vi "GetSortedPanes.vi"(8 "error in (no error)":errorcluster, 11 "Panes[]":refnum<vi>[](array[refnum])) -> (0 "error out":errorcluster, 3 "Panes":T1)   [LabVIEW 2022 SP3, in "PentaPanesLibrary.lvlib" / "PentaPanes.lvclass"]
uses:
  PentaPanes.lvclass
  PanesCluster.ctl
panel:
  out "Array":string[](array[string])
  out "appended array":refnum<vi>[](array[refnum])
  out "Center Index":i32
  out "Top Index":i32
  out "Bottom Index":i32
  out "Left Index":i32
  out "Right index":i32
  out "Vertical Center of panes":dbl[](array[numeric])
  out "Horizontal Center of pane":dbl[](array[numeric])
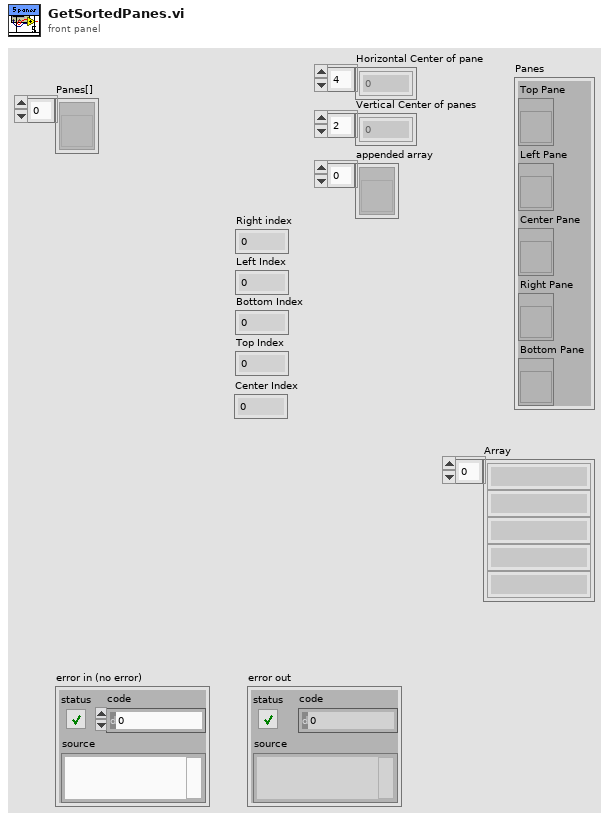
[diagram p1: front panel]
types:
  T1 = typedef "PentaPanesLibrary.lvlib/PentaPanes.lvclass/PanesCluster.ctl" = cluster{"Top Pane":refnum<vi>, "Left Pane":refnum<vi>, "Center Pane":refnum<vi>, "Right Pane":refnum<vi>, "Bottom Pane":refnum<vi>}
  T2 = typedef "LVPointTypeDef.ctl" = cluster{"Horizontal":i16, "Vertical":i16}
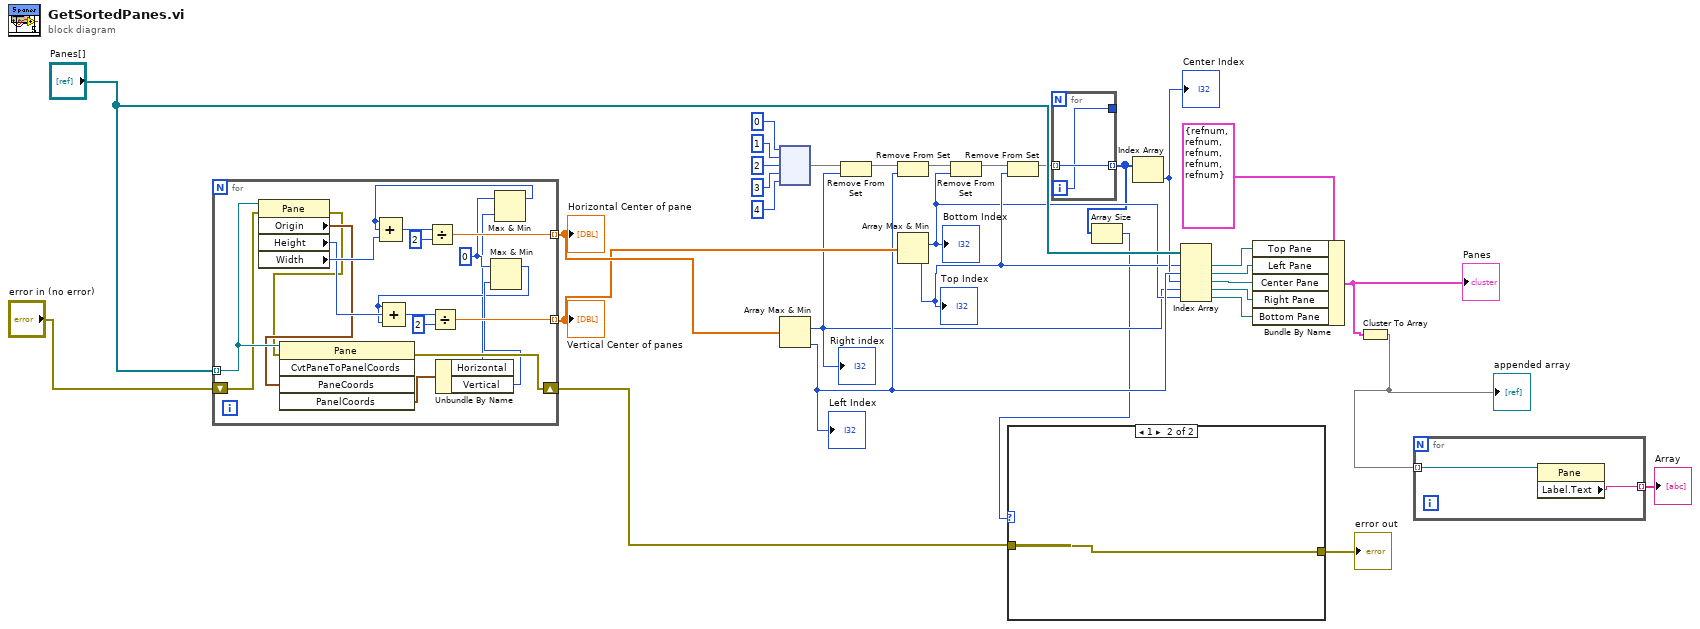
[diagram p0: block diagram]
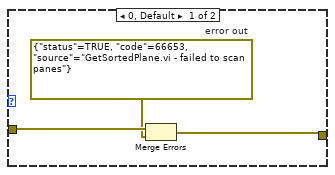
[diagram p2: hidden frame]
diagram:
  n1 = for {
    tunnel: "Panes[]" -> [w43] mode=indexing
    tunnel: [w45] -> w31 mode=indexing
    tunnel: [w44] -> w32 mode=indexing
    shift-right: [w38] -> w3
    shift-left: "error in (no error)" -> [w40]
    w35 = i16 0 ("x")
    n2 = property class="Pane"(reference=w43, error in=w40) -> (error out=w39:errorcluster, "Origin"=w42:T2, "Height"=w46:u32, "Width"=w51:u32)  [unwired: 1 out]
    n3 = invoke class="Pane" method="CvtPaneToPanelCoords"(reference=w43, error in=w39, "PaneCoords"=w42) -> (error out=w38:errorcluster, "PanelCoords"=w41:T2)  [unwired: 2 in, 3 out]
    n4 = Unbundle By Name(w41) -> ("Horizontal"=w34:i16, "Vertical"=w37:i16)
    n5 = Max & Min(x=w35, y=w37) -> (max(x,y)=w36:i16)  [unwired: 1 out]
    n6 = Compound Arithmetic op=ADD(w36, w46, w36) -> (w48:u32)
    n7 = Divide(x=w48, y=u32 2) -> (x/y=w45:dbl)
    n8 = Max & Min(x=w35, y=w34) -> (max(x,y)=w33:i16)  [unwired: 1 out]
    n9 = Compound Arithmetic op=ADD(w33, w33, w51) -> (w50:u32)
    n10 = Divide(x=w50, y=u32 2) -> (x/y=w44:dbl)
  }
  "Horizontal Center of pane" <- w32
  "Vertical Center of panes" <- w31
  n11 = node(0, 1 ("element"), 2 ("element"), 3 ("element"), 4 ("element")) -> (w6:set{i32})
  n12 = Array Max & Min(array=w32) -> (max index (indices)=w7:i32, min index (indices)=w23:i32)  [unwired: 2 out]
  "Right index" <- w7
  "Left Index" <- w23
  n13 = Remove From Set(10:w7, 11:w6) -> (3:w24:set{i32})  [unwired: 1 out]
  n14 = Remove From Set(10:w23, 11:w24) -> (3:w22:set{i32})  [unwired: 1 out]
  n15 = Array Max & Min(array=w31) -> (max index (indices)=w8:i32, min index (indices)=w9:i32)  [unwired: 2 out]
  "Bottom Index" <- w8
  "Top Index" <- w9
  n16 = Remove From Set(10:w8, 11:w22) -> (3:w21:set{i32})  [unwired: 1 out]
  n17 = Remove From Set(10:w9, 11:w21) -> (3:w18:set{i32})  [unwired: 1 out]
  n18 = for {
    tunnel: [w53] -> w5 mode=indexing
    tunnel: w18 -> [w53] mode=indexing
    tunnel: [w52] -> _
    i -> [w52]
  }
  n19 = Array Size(array=w5) -> (size(s)=w4:i32)
  n20 = case shown="1" w4 {
    tunnel: w3 -> [w56 w57]
    tunnel: [w54 w57] -> w2
    frame 0, Default {
      w55 = errorcluster {"status"=TRUE, "code"=66653, "source"="GetSortedPlane.vi - failed to scan panes"}  # error out
      n21 = Merge Errors(w56, w55) -> (w54:errorcluster)
    }
    frame 1 {
    }
  }
  "error out" <- w2
  n22 = Index Array(array=w5) -> (element=w20:i32)  [unwired: 1 in]
  "Center Index" <- w20
  n23 = Index Array(array="Panes[]", index #1=w9, index #2=w23, index #3=w20, index #4=w7, index #5=w8) -> (element #1=w16:refnum<vi>, element #2=w15:refnum<vi>, element #3=w14:refnum<vi>, element #4=w13:refnum<vi>, element #5=w12:refnum<vi>)
  n24 = Bundle By Name(cluster=T1 {"Top Pane"=refnum, "Left Pane"=refnum, "Center Pane"=refnum, "Right Pane"=refnum, "Bottom Pane"=refnum} ("Panes"), "Top Pane"=w16, "Left Pane"=w15, "Center Pane"=w14, "Right Pane"=w13, "Bottom Pane"=w12) -> (w11:T1)
  "Panes" <- w11
  n25 = Cluster To Array(cluster=w11) -> (array=w1:refnum<vi>[])
  "appended array" <- w1
  n26 = for {
    tunnel: w1 -> [w59] mode=indexing
    tunnel: [w58] -> w10 mode=indexing
    n27 = property class="Pane"(reference=w59) -> ("Label.Text"=w58:string)  [unwired: 1 in, 2 out]
  }
  "Array" <- w10
